vi "ESP300Write2.vi"(4 "error in (no error)":errorcluster, 5 "Command":string, 6 "ESP300 Channel":string, 7 "ESP300 Address":string) -> (0 "error out":errorcluster)   [LabVIEW 2010]
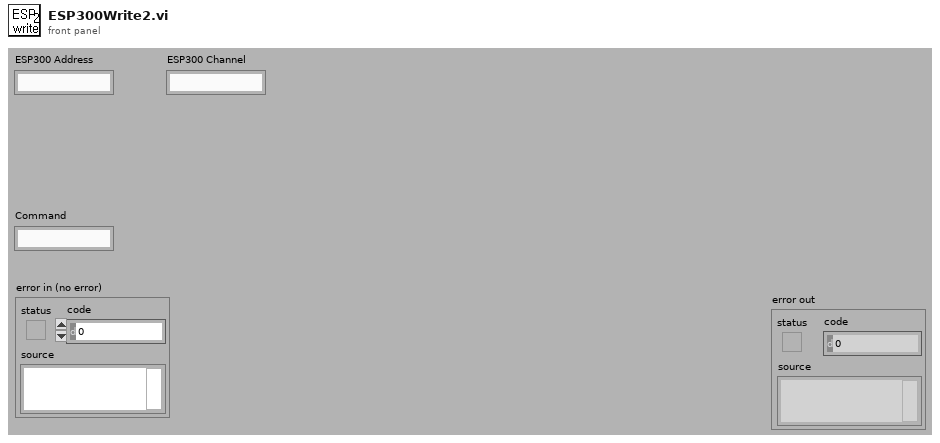
[diagram p1: front panel]
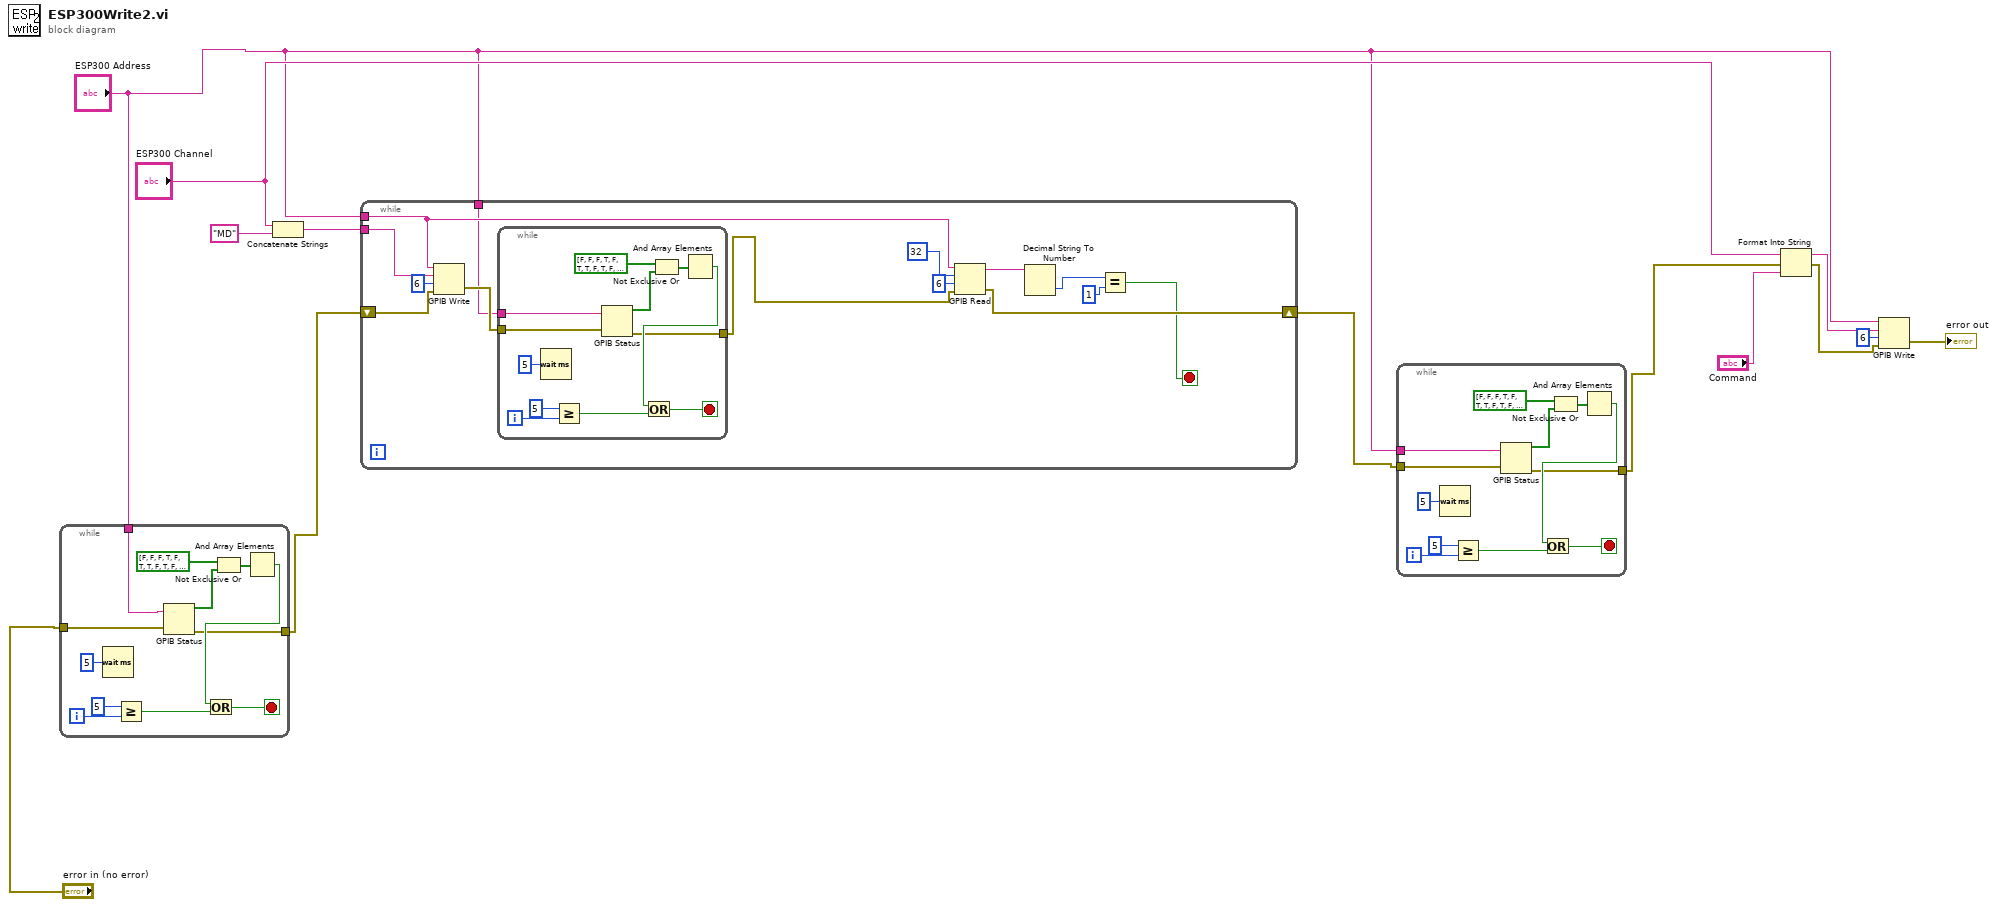
[diagram p0: block diagram]
diagram:
  n1 = while {
    tunnel: "error in (no error)" -> [w25]
    tunnel: [w15] -> w4
    tunnel: "ESP300 Address" -> [w14]
    i -> [w24]
    stop <- w21 stop-if-true
    n2 = Wait (ms)(milliseconds to wait=u32 5) -> ()  [unwired: 1 out]
    n3 = Greater Or Equal?(x=5, y=w24) -> (x >= y?=w22:bool)
    n4 = GPIB Status(0:w14, 1:w25) -> (2:w19:bool[], 5:w15:errorcluster)  [unwired: 2 out]
    n5 = Not Exclusive Or(1:w19, 2:bool[] [FALSE, FALSE, FALSE, TRUE, FALSE, TRUE, TRUE, FALSE, TRUE, FALSE, FALSE, FALSE, FALSE, FALSE, FALSE, FALSE] ("status 2")) -> (0:w18:bool[])
    n6 = And Array Elements(Boolean array=w18) -> (logical AND=w17:bool)
    n7 = Or(x=w17, y=w22) -> (x .or. y?=w21:bool)
  }
  n8 = Concatenate Strings("ESP300 Channel", "MD" ("string")) -> (w10:string)
  n9 = while {
    tunnel: w10 -> [w39]
    tunnel: "ESP300 Address" -> [w36]
    shift-right: [w34] -> w3
    shift-left: w4 -> [w37]
    tunnel: "ESP300 Address" -> [w26]
    stop <- w30 stop-if-true
    n10 = GPIB Write(0:w36, 1:w39, 2:i16 6 ("mode (0)"), 3:w37) -> (6:w28:errorcluster)  [unwired: 1 in, 1 out]
    n11 = while {
      tunnel: w28 -> [w51]
      tunnel: [w41] -> w27
      tunnel: w26 -> [w40]
      i -> [w50]
      stop <- w47 stop-if-true
      n12 = Wait (ms)(milliseconds to wait=u32 5) -> ()  [unwired: 1 out]
      n13 = Greater Or Equal?(x=5, y=w50) -> (x >= y?=w48:bool)
      n14 = GPIB Status(0:w40, 1:w51) -> (2:w45:bool[], 5:w41:errorcluster)  [unwired: 2 out]
      n15 = Not Exclusive Or(1:w45, 2:bool[] [FALSE, FALSE, FALSE, TRUE, FALSE, TRUE, TRUE, FALSE, TRUE, FALSE, FALSE, FALSE, FALSE, FALSE, FALSE, FALSE] ("status 2")) -> (0:w44:bool[])
      n16 = And Array Elements(Boolean array=w44) -> (logical AND=w43:bool)
      n17 = Or(x=w43, y=w48) -> (x .or. y?=w47:bool)
    }
    n18 = GPIB Read(0:w36, 1:32 ("byte count"), 2:i16 6 ("mode (0)"), 3:w27) -> (5:w33:string, 7:w34:errorcluster)  [unwired: 1 in, 1 out]
    n19 = Decimal String To Number(string=w33) -> (number=w32:i32)  [unwired: 2 in, 1 out]
    n20 = Equal?(x=w32, y=1) -> (x = y?=w30:bool)
  }
  n21 = while {
    tunnel: w3 -> [w63]
    tunnel: [w53] -> w2
    tunnel: "ESP300 Address" -> [w52]
    i -> [w62]
    stop <- w59 stop-if-true
    n22 = Wait (ms)(milliseconds to wait=u32 5) -> ()  [unwired: 1 out]
    n23 = Greater Or Equal?(x=5, y=w62) -> (x >= y?=w60:bool)
    n24 = GPIB Status(0:w52, 1:w63) -> (2:w57:bool[], 5:w53:errorcluster)  [unwired: 2 out]
    n25 = Not Exclusive Or(1:w57, 2:bool[] [FALSE, FALSE, FALSE, TRUE, FALSE, TRUE, TRUE, FALSE, TRUE, FALSE, FALSE, FALSE, FALSE, FALSE, FALSE, FALSE] ("status 2")) -> (0:w56:bool[])
    n26 = And Array Elements(Boolean array=w56) -> (logical AND=w55:bool)
    n27 = Or(x=w55, y=w60) -> (x .or. y?=w59:bool)
  }
  n28 = Format Into String(initial string="ESP300 Channel", error in=w2, "Command") -> (resulting string=w12:string, error out=w8:errorcluster)  [unwired: 1 in]
  n29 = GPIB Write(0:"ESP300 Address", 1:w12, 2:i16 6 ("mode (0)"), 3:w8) -> (6:→"error out":errorcluster)  [unwired: 1 in, 1 out]
